vi "LTVDiffDriveCtrl_SetTolerance.vi"(8 "RightVelTolerance":dbl, 9 "LeftVelTolerance":dbl, 10 "PoseTolerance":T1={"TRANSLATION"={"X"=0.0, "Y"=0.0}, "ROTATION"={"VALUE"=0.0, "COS"=1.0, "SIN"=0.0}} {"ROTATION"."SIN" format="%13.4f"; "ROTATION"."COS" format="%13.4f"; "ROTATION"."VALUE" format="%13.4f"; "TRANSLATION"."Y" format="%14.3f"; "TRANSLATION"."X" format="%14.3f"}, 11 "in LTV_DIFF_DRIVE_CONTROLLER":T4) -> (3 "out LTV_DIFF_DRIVE_CONTROLLER":T4)   [LabVIEW 2019, in "Trajectory_Library.lvlib"]
doc: "Create implicit model follower\n\nInputs:\n - A < states, states > -- Continuous system matrix of the plant being controlled.\n - B < states, inputs > -- Continuous input matrix of the plant being controlled.\n - A_Ref < states, states > -- Continuous system matrix whose dymanics should be followed.\n - B_Ref < states, inputs > -- Continuous input matrix x whose dymanics should be followed.\n\nOutputs:\n - Error -- If TRUE, an error occured."
uses:
  <vilib>/Analysis/Matrix/Datatypes/RealMatrix.ctl
  POSE2D.ctl
  TRANSLATION2D.ctl
  ROTATION2D.ctl
  Trajectory_Library.lvlib
  <vilib>/Analysis/Matrix/NI_Matrix.lvlib
  FUNCTION_GENERATOR_MATRIX.ctl
  LTV_DIFF_DRIVE_CTRL.ctl
panel:
  # "< 5, 1 >"
  # "< 5, 1 >"
  # "< 5, 1 >"
  # "< 5, 1 >"
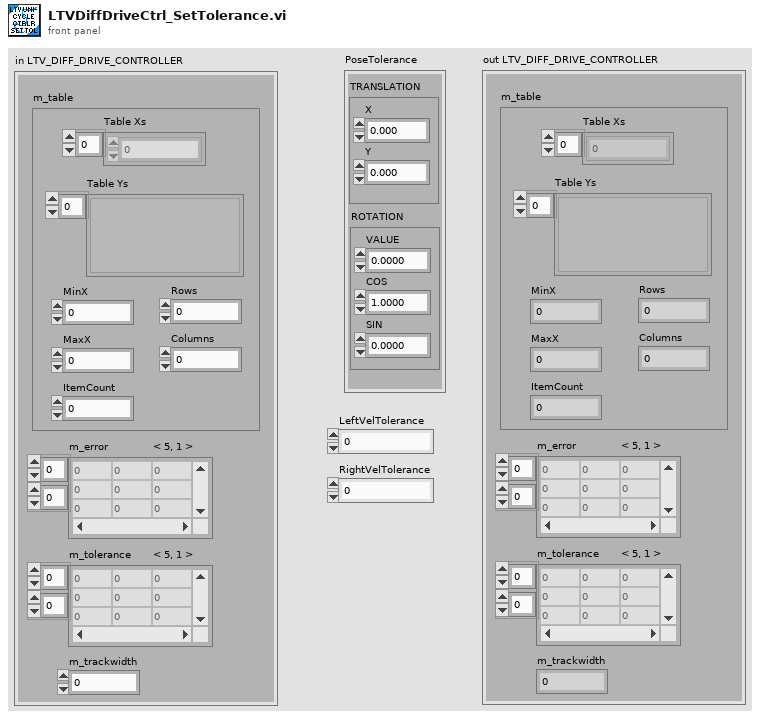
[diagram p1: front panel]
types:
  T1 = typedef "Trajectory_Library.lvlib/POSE2D.ctl" = cluster{"TRANSLATION":T2, "ROTATION":T3}
  T2 = typedef "Trajectory_Library.lvlib/TRANSLATION2D.ctl" = cluster{"X":dbl, "Y":dbl}
  T3 = typedef "Trajectory_Library.lvlib/ROTATION2D.ctl" = cluster{"VALUE":dbl, "COS":dbl, "SIN":dbl}
  T4 = typedef "Trajectory_Library.lvlib/LTV_DIFF_DRIVE_CTRL.ctl" = cluster{"m_table":T5, "m_error":T6, "m_tolerance":T6, "m_trackwidth":dbl}
  T5 = typedef "Trajectory_Library.lvlib/FUNCTION_GENERATOR_MATRIX.ctl" = cluster{"Table Xs":dbl[], "Table Ys":variant[], "MinX":dbl, "MaxX":dbl, "ItemCount":i32, "Rows":i32, "Columns":i32}
  T6 = typedef "NI_Matrix.lvlib/RealMatrix.ctl" = dbl[][]
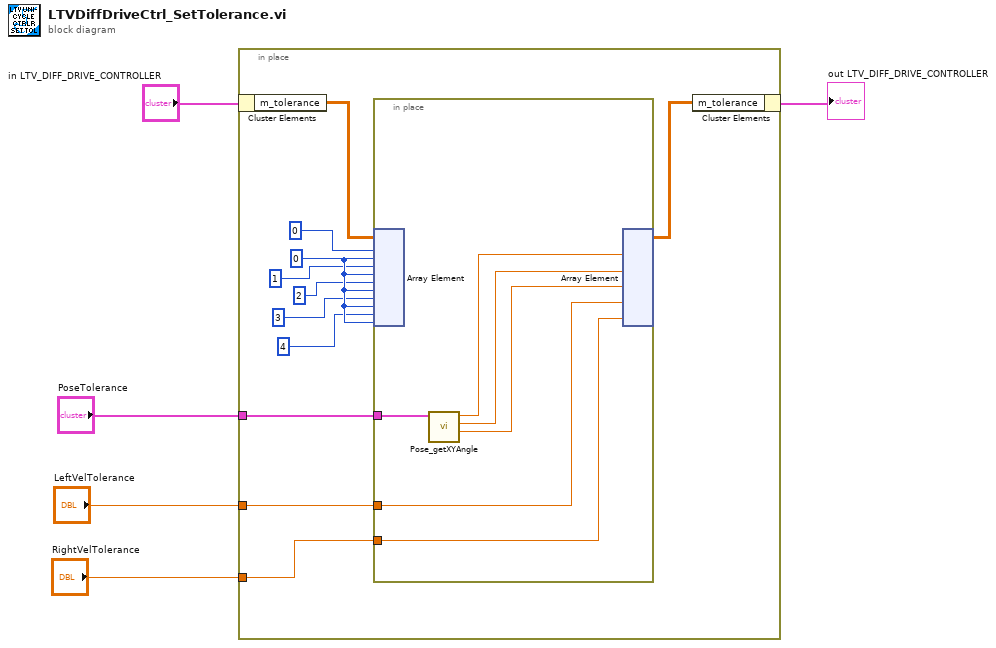
[diagram p0: block diagram]
diagram:
  n1 = in-place {
    in-place-border: "PoseTolerance" -> [w6]
    in-place-border: "RightVelTolerance" -> [w15]
    in-place-border: "LeftVelTolerance" -> [w7]
    w13 = 0
    n2 = in-place-cluster #1("in LTV_DIFF_DRIVE_CONTROLLER") -> ("m_tolerance"=w16:T6)
    n3 = in-place {
      in-place-border: w15 -> [w22]
      in-place-border: w7 -> [w21]
      in-place-border: w6 -> [w20]
      n4 = in-place-array #2(w16, 0, w13, 1, w13, 2, w13, 3, w13, 4, w13) -> ()  [unwired: 5 out]
      n5 = call "Pose_getXYAngle.vi"("in POSE"=w20) -> ("Angle"=w17:dbl, "Y"=w18:dbl, "X"=w19:dbl)  [unwired: 8 in]
      n6 = in-place-array #2(w19, w18, w17, w21, w22) -> (w8:T6)  [unwired: 10 out]
    }
    n7 = in-place-cluster #1("m_tolerance"=w8) -> (→"out LTV_DIFF_DRIVE_CONTROLLER":T4)
  }
